vi "Dispose Table.vi"(8 "error in (no error)":errorcluster caption="错误输入（无错误）", 11 "DataTable 输入":refnum<class "DataTable.lvclass"> caption="DNL_LabVIEW Object in") -> (0 "error out":errorcluster caption="错误输出", 3 "DataTable 输出":refnum<class "DataTable.lvclass"> caption="DNL_LabVIEW Object out")   [LabVIEW 2012, in "Data Grid VIEW.lvlib" / "DataTable.lvclass"]
uses:
  DataTable.lvclass
  DataTable.lvclass/DataTable.ctl
  System.Data
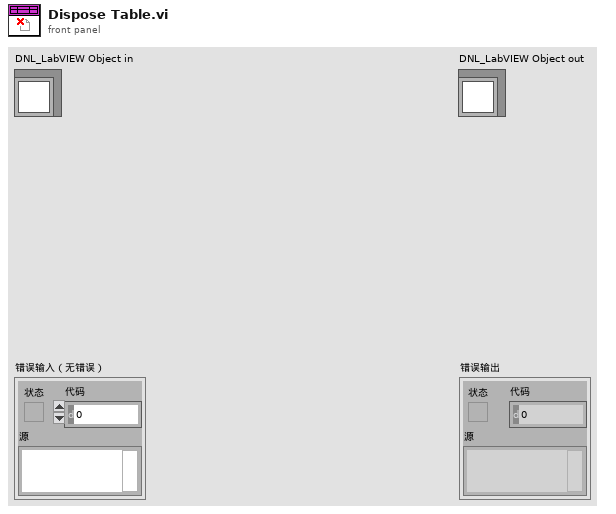
[diagram p1: front panel]
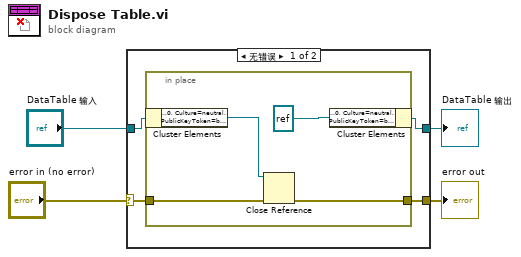
[diagram p0: block diagram]
diagram:
  n1 = case shown="无错误" "error in (no error)" {
    selector: "error in (no error)" -> [w7 w14]
    tunnel: [w6 w14] -> w3
    tunnel: [w5 w13] -> w1
    tunnel: "DataTable 输入" -> [w8 w13]
    frame No Error {
      n2 = in-place {
        in-place-border: w7 -> [w9]
        in-place-border: [w11] -> w6
        n3 = in-place-cluster #1(w8) -> ("DataTable"=w12:refnum<k24>)
        n4 = Close Reference(reference=w12, error in (no error)=w9) -> (error out=w11:errorcluster)
        n5 = in-place-cluster #1("DataTable"=refnum<k24> refnum) -> (w5:refnum<class "DataTable.lvclass">)
      }
    }
    frame Error {
    }
  }
  "error out" <- w3
  "DataTable 输出" <- w1
